vi "Focus.vi"() -> ()   [LabVIEW 2013]
panel:
  out "?":u16[](graph)
  in  "Colum of interest":i32
  in  "Raw of interesr":i32
  out "?":u16[](graph)
  in  "stop":bool
  out "Intensity Graph":u16[][](graph)
  in  "Exposure":dbl=0.001 format="%.3f"
  in  "Close Compensation time ms 2":u32=8
  in  "Open Compensation time ms":u32=8
  in  "Temperature":dbl format="%.2f"
  out "error out":errorcluster
  in  "error in (no error)":errorcluster
  # "Note: for the Cascade and PhotonMax\nthe open/close compensation should be 0"
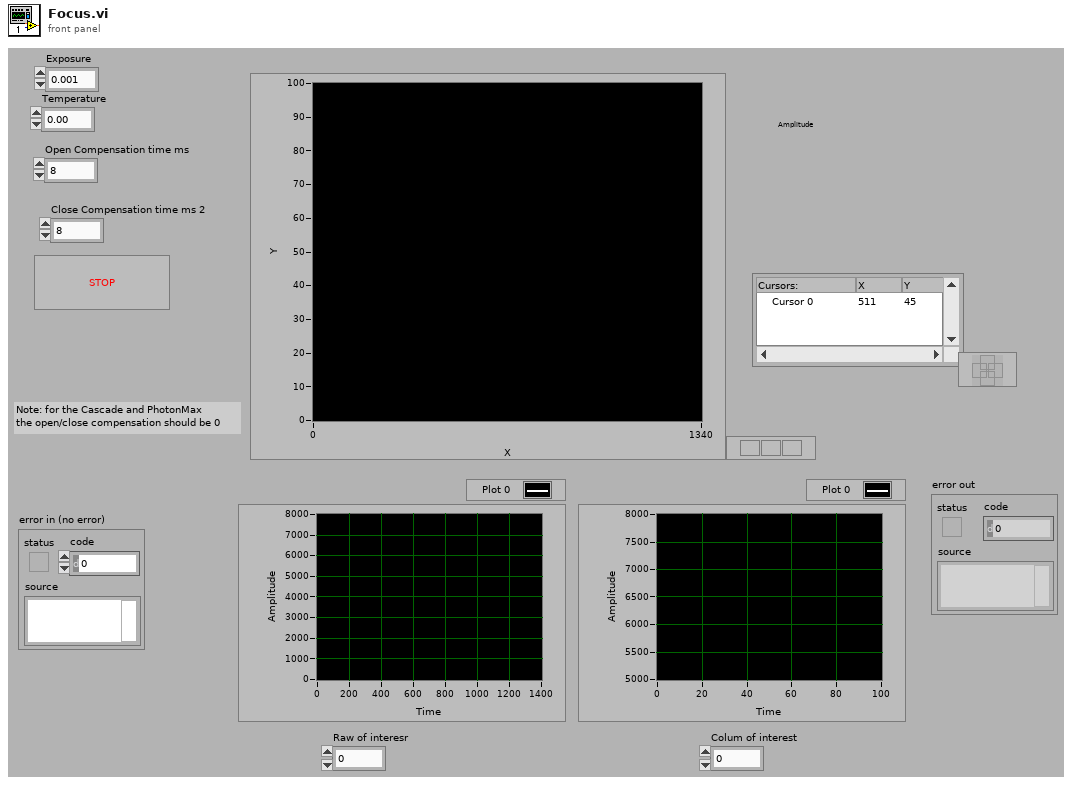
[diagram p1: front panel]
types:
  T1 = cluster{"Open Compensation time ms":u32, "Close Compensation time ms 2":u32}
  T2 = cluster{"Camera Handle":u32, "File Handle":u32, "Image Handle":u32}
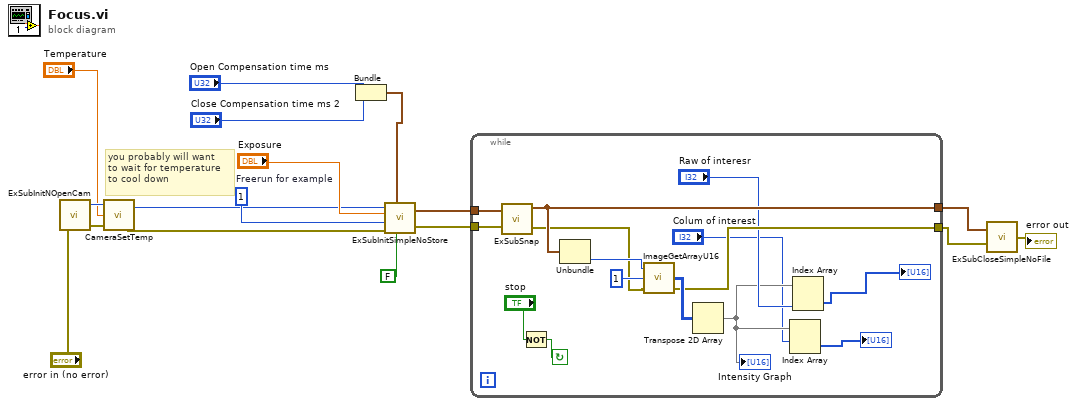
[diagram p0: block diagram]
diagram:
  w4 = 1  # Freerun for example
  # "you probably will want \nto wait for temperature \nto cool down"
  n1 = call "ExSubInitNOpenCam.vi"("error in (no error)"="error in (no error)") -> ("Camera Handle"=w15:u32, "error out"=w16:errorcluster)
  n2 = call <userlib>:"CameraSetTemp.vi"("error in (no error)"=w16, "Temperature"="Temperature", "Camera Handle"=w15) -> ("error out"=w10:errorcluster, "Camera Handle"=w3:u32)
  n3 = Bundle("Open Compensation time ms"="Open Compensation time ms", "Close Compensation time ms 2"="Close Compensation time ms 2") -> (w7:T1)  [unwired: 1 in]
  n4 = call "ExSubInitSimpleNoStore.vi"("Intensifier"=FALSE, "Shutter Comp"=w7, "error in (no error)"=w10, "Triggering mode"=w4, "Exposure"="Exposure", "Camera Handle"=w3) -> ("error out"=w11:errorcluster, "Handles"=w12:cluster{"Camera":u32, "File":u32, "Image":u32})
  n5 = while {
    tunnel: w12 -> [w32]
    tunnel: w11 -> [w31]
    tunnel: [w26] -> w2
    tunnel: [w23] -> w1
    stop <- w30 continue-if-true
    n6 = call "ExSubSnap.vi"("error in (no error)"=w31, "Handle Cluster"=w32) -> ("error out"=w24:errorcluster, "Handle Cluster Out"=w26:T2)
    n7 = Not(x="stop") -> (.not. x?=w30:bool)
    n8 = Unbundle(w26) -> ("Image Handle"=w25:u32)  [unwired: 2 out]
    n9 = call <userlib>:"ImageGetArrayU16.vi"("error in"=w24, "Z position"=1, "Image Handle"=w25) -> ("error out"=w23:errorcluster, "Array uint 16"=w28:u16[][])  [unwired: 1 out]
    n10 = Transpose 2D Array(2D array=w28) -> (transposed array=w21:u16[][])
    "Intensity Graph" <- w21
    n11 = Index Array(array=w21, index (row)="Colum of interest") -> (element=→"?":u16[])  [unwired: 1 in]
    n12 = Index Array(array=w21, index (col)="Raw of interesr") -> (element=→"?":u16[])  [unwired: 1 in]
  }
  n13 = call "ExSubCloseSimpleNoFile.vi"("error in (no error)"=w1, "Handles In"=w2) -> ("error out"=→"error out":errorcluster)
